vi "Lissajous.vi"() -> ()   [LabVIEW 2016]
uses:
  Biblioteca.lvlib
panel:
  in  "Pausa":bool
  out "Y2":dbl[](graph)
  out "Y1":dbl[](graph)
  in  "B":dbl=1.0
  in  "A":dbl=1.0
  in  "w2":dbl=4.0
  in  "Q":dbl=1.57
  in  "w1":dbl=3.0
  in  "Parar":bool
  out "XY Graph":cluster{dbl[], dbl[]}(graph)
  # "Experimentação com Figuras de Lissajous"
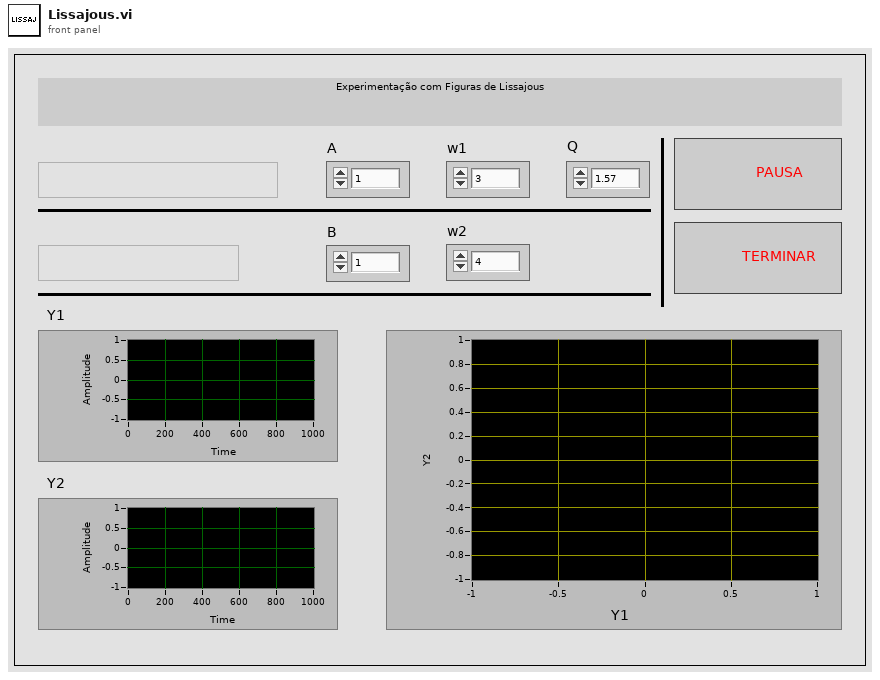
[diagram p1: front panel]
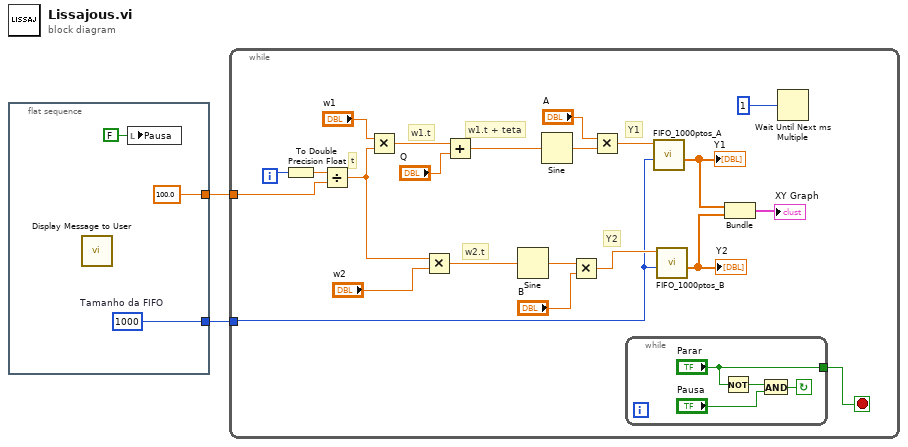
[diagram p0: block diagram]
diagram:
  n1 = flat-sequence {
    tunnel: [100.0 ("y")] -> w2
    tunnel: [w3] -> w1
    frame #0 {
      w3 = 1000  # Tamanho da FIFO
      n2 = call "Display Message to User"() -> ()  [unwired: 10 in, 2 out]
      n3 = local write "Pausa"(FALSE ("Pausa")) -> ()
    }
  }
  n4 = while {
    tunnel: w2 -> [w10]
    tunnel: w1 -> [w9]
    i -> [w19]
    stop <- w6 stop-if-true
    # "Y2"
    # "Y1"
    # "w1.t + teta"
    # "w2.t"
    # "w1.t"
    # "t"
    n5 = To Double Precision Float(number=w19) -> (double precision float=w20:dbl)
    n6 = Divide(x=w20, y=w10) -> (x/y=w16:dbl)
    n7 = Multiply(x="w1", y=w16) -> (x*y=w25:dbl)
    n8 = Multiply(x=w16, y="w2") -> (x*y=w21:dbl)
    n9 = Add(x=w25, y="Q") -> (x+y=w24:dbl)
    n10 = Sine(x=w21) -> (sin(x)=w7:dbl)
    n11 = Sine(x=w24) -> (sin(x)=w26:dbl)
    n12 = Multiply(x=w7, y="B") -> (x*y=w15:dbl)
    n13 = Multiply(x="A", y=w26) -> (x*y=w12:dbl)
    n14 = while {
      tunnel: ["Parar"] -> w6
      stop <- w30 continue-if-true
      n15 = Not(x="Parar") -> (.not. x?=w29:bool)
      n16 = And(x=w29, y="Pausa") -> (x .and. y?=w30:bool)
    }
    n17 = call "FIFO_1000ptos_A.vi"("Tamanho da FIFO"=w9, "Valor_Entrada"=w12) -> ("Array"=w11:dbl[])  [unwired: 8 in, 1 out]
    "Y1" <- w11
    n18 = call "FIFO_1000ptos_B.vi"("Tamanho da FIFO"=w9, "Valor_Entrada"=w15) -> ("Array"=w14:dbl[])  [unwired: 8 in, 1 out]
    "Y2" <- w14
    n19 = Bundle("Array"=w11, "Array"=w14) -> (→"XY Graph":cluster{"Array":dbl[], "Array":dbl[]})  [unwired: 1 in]
    n20 = Wait Until Next ms Multiple(millisecond multiple=u32 1 ("milliseconds to wait")) -> ()  [unwired: 1 out]
  }
